vi "KeithleyTDS.vi"() -> ()   [LabVIEW 2014]
doc: "Configures a sweep and takes voltage and current readings at each point."
uses:
  <vilib>/Analysis/1siggen.llb/Ramp Pattern by Samples.vi
  <instrlib>/Keithley 24XX/Public/Data/Read (Single Point).vi
  <vilib>/Waveform/WDTFileIO.llb/Export Waveform To Spreadsheet File.vi
  <instrlib>/Tektronix TDS 200 1000 2000 Series/Tektronix TDS 200 1000 2000 Series.lvlib
  <instrlib>/Keithley 24XX/Keithley 24XX.lvlib
  <vilib>/Analysis/NI_AALBase.lvlib
panel:
  out "Current":sgl
  out "Voltage":string
  in  "Vmax":dbl
  in  "Source Mode  (0: Voltage)":u16(ring) items=["Voltage", "Current"]
  in  "Compliance  Level (0.1)":dbl=0.1
  in  "Vmin":dbl
  in  "Enable Current Auto Range (T:Enable)":bool=TRUE
  in  "Current Manual Range (1.0)":dbl=1.0
  in  "Serial Keithley":T1={"Baud Rate"=9600, "Parity"=0, "Data Bits"=8, "Stop Bits"=10, "Flow Control"=0} {"Flow Control" items=["None", "XON/XOFF", "RTS/CTS", "XON/XOFF & RTS/CTS", "DTR/DSR", "XON/XOFF & DTR/DSR"]; "Stop Bits" items=["1.0"=10, "1.5"=15, "2.0"=20]; "Data Bits" items=["7"=7, "8"=8]; "Parity" items=["None", "Odd", "Even", "Mark", "Space"]; "Baud Rate" items=["300"=300, "600"=600, "1200"=1200, "2400"=2400, "4800"=4800, "9600"=9600, "19200"=19200]}
  in  "VISA resource Keithley":refnum<visa-resource-name>
  out "FilePath":path
  in  "Number of Points":dbl
  in  "Serial TDS":T2={"Baud Rate"=9600, "Parity"=0, "Stop Bits"=10, "Flow Control"=0} {"Flow Control" items=["None", "XON/XOFF", "RTS/CTS", "XON/XOFF & RTS/CTS", "DTR/DSR", "XON/XOFF & DTR/DSR"]; "Stop Bits" items=["1.0"=10, "1.5"=15, "2.0"=20]; "Parity" items=["None", "Odd", "Even", "Mark", "Space"]; "Baud Rate" items=["300"=300, "600"=600, "1200"=1200, "2400"=2400, "4800"=4800, "9600"=9600, "19200"=19200]}
  in  "VISA resource TDS":refnum<visa-resource-name>
  in  "TimeDelay (ms)":dbl
  in  "Source (0: Channel 1)":u16(ring) items=["Channel 1", "Channel 2", "Channel 3", "Channel 4", "Math", "Reference A", "Reference B", "Reference C", "Reference D", "FFT"]
  in  "Timeout (10000 ms)":u32=10000
  out "Waveform Data":waveform(dbl)(graph)
  out "error out":errorcluster
  # "(c) 2006 - 2011 National Instruments.  ALL RIGHTS RESERVED."
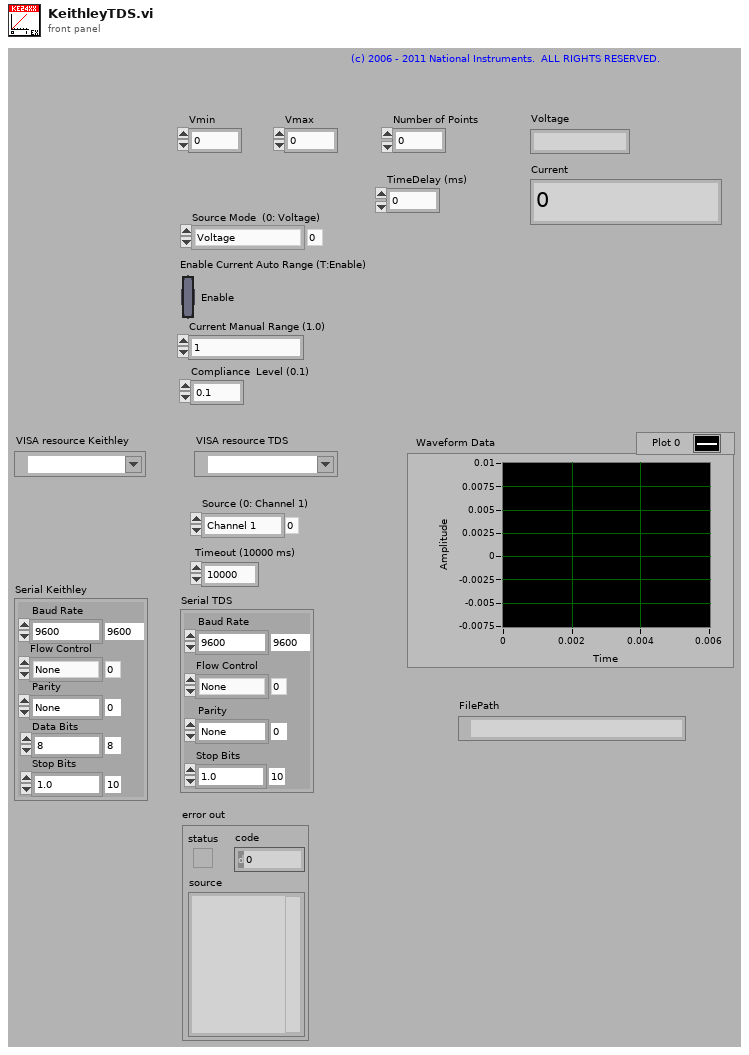
[diagram p1: front panel]
types:
  T1 = cluster{"Baud Rate":u32, "Parity":u16, "Data Bits":u16, "Stop Bits":u16, "Flow Control":u16}
  T2 = cluster{"Baud Rate":u32, "Parity":u16, "Stop Bits":u16, "Flow Control":u16}
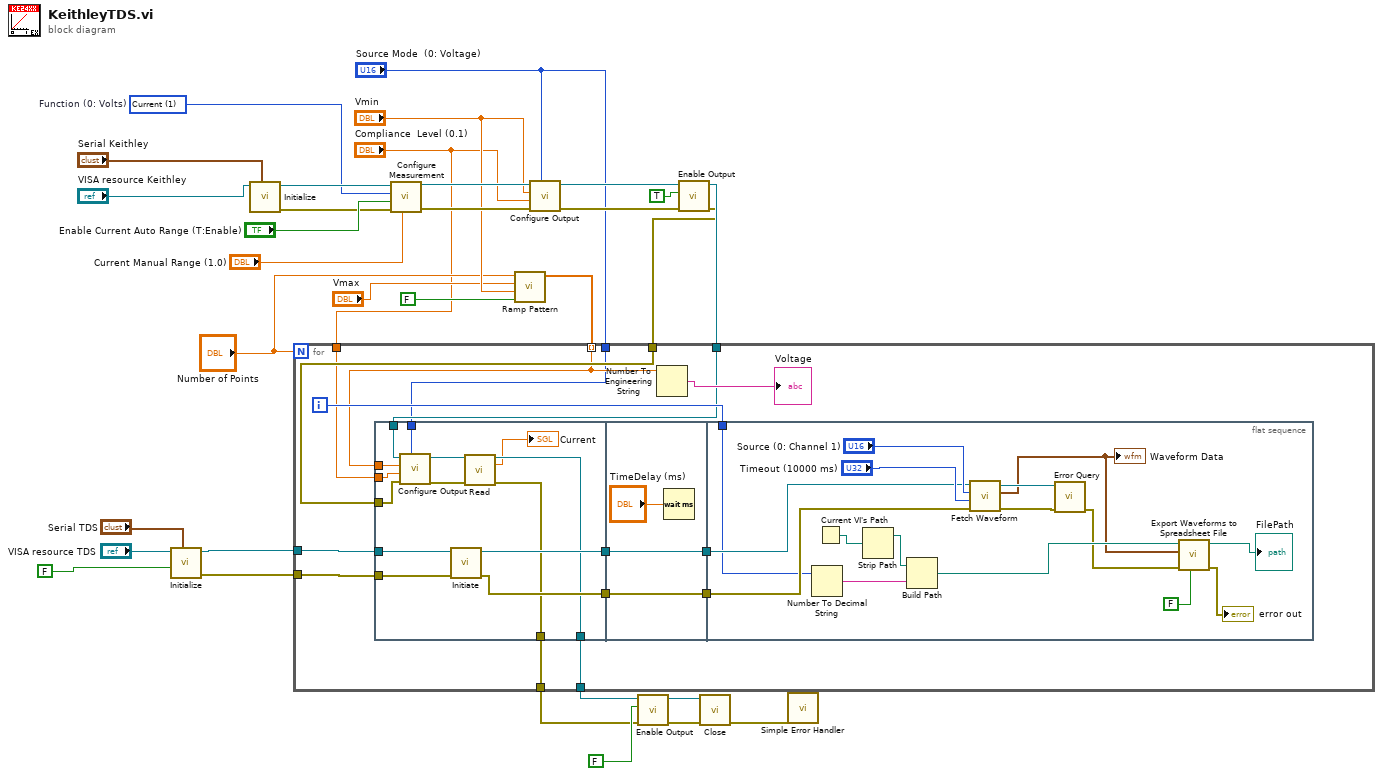
[diagram p0: block diagram]
diagram:
  w20 = u16 1 items=["Volts", "Current", "Resistance"]  # Function (0: Volts)
  n1 = call <instrlib>:"Initialize.vi"("Serial Configuration"="Serial TDS", "Reset? (T: Yes)"=FALSE, "VISA resource name"="VISA resource TDS") -> ("error out"=w28:errorcluster, "VISA resource name out"=w29:refnum<visa-resource-name>)  [unwired: 2 in, 5 out]
  n2 = call <instrlib>:"Initialize.vi"("Serial Configuration"="Serial Keithley", "VISA resource name"="VISA resource Keithley") -> ("error out"=w22:errorcluster, "VISA resource name out"=w21:refnum<visa-resource-name>)  [unwired: 8 in]
  n3 = call <instrlib>:"Configure Measurement.vi"("Manual Range (1.0)"="Current Manual Range (1.0)", "error in (no error)"=w22, "Enable Auto Range (T:Enable)"="Enable Current Auto Range (T:Enable)", "Function (0: Volts)"=w20, "VISA resource name"=w21) -> ("error out"=w18:errorcluster, "VISA resource name out"=w19:refnum<visa-resource-name>)  [unwired: 5 in]
  n4 = call-poly <vilib>:"Ramp Pattern.vi"("exclude end?"=FALSE, "start"="Vmin", "end"="Vmax", "samples"="Number of Points") -> ("Ramp Pattern"=w11:dbl[])  [unwired: 6 in, 1 out]
  n5 = call <instrlib>:"Configure Output.vi"("Source Mode  (0: Voltage)"="Source Mode  (0: Voltage)", "error in (no error)"=w18, "Compliance  Level (0.1)"="Compliance  Level (0.1)", "Output Level (0)"="Vmin", "VISA resource name"=w19) -> ("error out"=w17:errorcluster, "VISA resource name out"=w16:refnum<visa-resource-name>)  [unwired: 5 in]
  n6 = call <instrlib>:"Enable Output.vi"("error in (no error)"=w17, "Enable Output (T: Enable)"=TRUE, "VISA resource name"=w16) -> ("error out"=w9:errorcluster, "VISA resource name out"=w10:refnum<visa-resource-name>)  [unwired: 7 in]
  n7 = for {
    N: "Number of Points" -> [_]
    tunnel: w29 -> [w43]
    tunnel: w28 -> [w42]
    tunnel: w11 -> [w37] mode=indexing
    tunnel: w10 -> [w39]
    tunnel: w9 -> [w38]
    tunnel: "Compliance  Level (0.1)" -> [w36]
    tunnel: "Source Mode  (0: Voltage)" -> [w35]
    tunnel: [w34] -> w5
    tunnel: [w33] -> w4
    i -> [w41]
    n8 = flat-sequence {
      tunnel: [w61] -> w47
      tunnel: [w60] -> w45
      tunnel: w43 -> [w59]
      tunnel: w42 -> [w58]
      tunnel: w39 -> [w57]
      tunnel: w38 -> [w56]
      tunnel: w37 -> [w55]
      tunnel: w36 -> [w54]
      tunnel: w35 -> [w51]
      tunnel: [w50] -> w34
      tunnel: [w49] -> w33
      tunnel: w47 -> [w63]
      tunnel: [w63] -> w46
      tunnel: w45 -> [w62]
      tunnel: [w62] -> w44
      tunnel: w46 -> [w75]
      tunnel: w44 -> [w76]
      tunnel: w41 -> [w71]
      frame #0 {
        n9 = call <instrlib>:"Configure Output.vi"("Source Mode  (0: Voltage)"=w51, "error in (no error)"=w56, "Compliance  Level (0.1)"=w54, "Output Level (0)"=w55, "VISA resource name"=w57) -> ("error out"=w52:errorcluster, "VISA resource name out"=w53:refnum<visa-resource-name>)  [unwired: 5 in]
        n10 = call <instrlib>:"Initiate.vi"("error in (no error)"=w58, "VISA resource name"=w59) -> ("error out"=w61:errorcluster, "VISA resource name out"=w60:refnum<visa-resource-name>)  [unwired: 8 out]
        n11 = call-poly <instrlib>:"Read.vi"("VISA resource name"=w53, "error in (no error)"=w52) -> ("VISA resource name out"=w49:refnum<visa-resource-name>, "Current"=→"Current":sgl, "error out"=w50:errorcluster)  [unwired: 7 in, 4 out]
      }
      frame #1 {
        n12 = Wait (ms)(milliseconds to wait="TimeDelay (ms)") -> ()  [unwired: 1 out]
      }
      frame #2 {
        n13 = Number To Decimal String(number=w71) -> (decimal integer string=w74:string)  [unwired: 1 in]
        n14 = Current VI's Path() -> (path=w73:path)
        n15 = Strip Path(path=w73) -> (stripped path=w72:path)  [unwired: 1 out]
        n16 = Build Path(base path=w72, name or relative path=w74) -> (appended path=w69:path)
        n17 = call <instrlib>:"Fetch Waveform.vi"("error in (no error)"=w75, "Timeout (10000 ms)"="Timeout (10000 ms)", "Source (0: Channel 1)"="Source (0: Channel 1)", "VISA resource name"=w76) -> ("error out"=w79:errorcluster, "Waveform Data"=w68:waveform(dbl), "VISA resource name out"=w80:refnum<visa-resource-name>)  [unwired: 2 in, 3 out]
        "Waveform Data" <- w68
        n18 = call <instrlib>:"Error Query.vi"("error in (no error)"=w79, "VISA resource name"=w80) -> ("error out"=w67:errorcluster)  [unwired: 9 out]
        n19 = call-poly <vilib>:"Export Waveforms to Spreadsheet File.vi"("append to file? (new file:F)"=FALSE, "error in (no error)"=w67, "waveform"=w68, "file path (dialog if empty)"=w69) -> ("error out"=→"error out":errorcluster, "new file path (Not A Path if cancelled)"=→"FilePath":path)  [unwired: 6 in]
      }
    }
    n20 = Number To Engineering String(4:w37) -> (0:→"Voltage":string)  [unwired: 3 in]
  }
  n21 = call <instrlib>:"Enable Output.vi"("error in (no error)"=w5, "Enable Output (T: Enable)"=FALSE, "VISA resource name"=w4) -> ("error out"=w2:errorcluster, "VISA resource name out"=w3:refnum<visa-resource-name>)  [unwired: 7 in]
  n22 = call <instrlib>:"Close.vi"("error in (no error)"=w2, "VISA resource name"=w3) -> ("error out"=w1:errorcluster)  [unwired: 9 in]
  n23 = call <vilib>:"Simple Error Handler.vi"("error in (no error)"=w1) -> ()  [unwired: 4 in, 5 out]
